vi "get remaining time budget.vi"(8 "error in":errorcluster, 10 "dt":u32=1, 11 "timing source in":refnum<class "scan engine timing source.lvclass">) -> (0 "error out":errorcluster, 2 "budget (ns)":u64, 3 "timing source out":refnum<class "scan engine timing source.lvclass">)   [LabVIEW 2013, in "scan engine timing source.lvclass"]
uses:
  scan engine timing source.lvclass
  scan engine timing source.lvclass/scan engine timing source.ctl
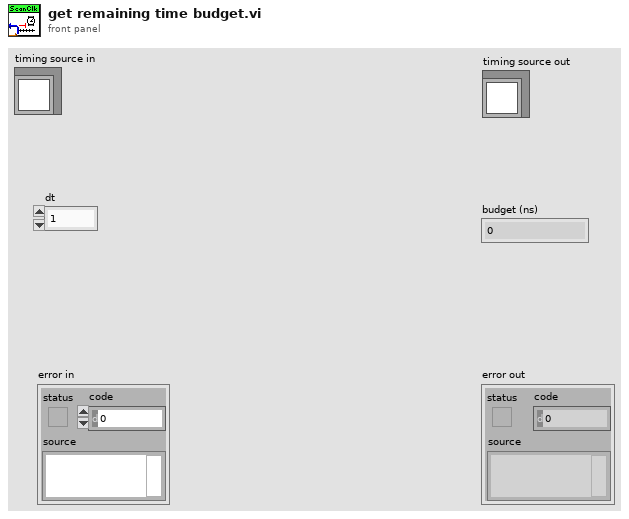
[diagram p1: front panel]
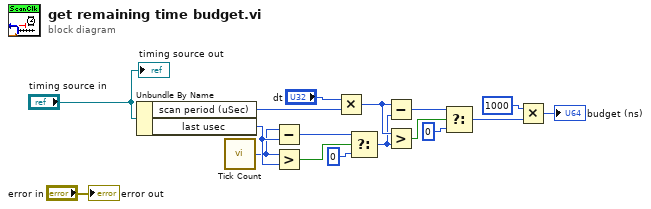
[diagram p0: block diagram]
diagram:
  n1 = Unbundle By Name("timing source in") -> ("scan period (uSec)"=w16:u32, "last usec"=w9:u32)
  n2 = call "Tick Count"() -> ("Tick Count(uSec)"=w8:u32)
  n3 = Subtract(x=w8, y=w9) -> (x-y=w11:u32)
  n4 = Greater?(x=w8, y=w9) -> (0:w12:bool)
  n5 = Multiply(x="dt", y=w16) -> (x*y=w4:u32)
  n6 = Select(t=w11, s=w12, f=u32 0) -> (s? t:f=w3:u32)
  n7 = Subtract(x=w4, y=w3) -> (x-y=w6:u32)
  n8 = Greater?(x=w4, y=w3) -> (0:w5:bool)
  n9 = Select(t=w6, s=w5, f=u32 0) -> (s? t:f=w2:u32)
  n10 = Multiply(x=u64 1000, y=w2) -> (x*y=→"budget (ns)":u64)
  "error out" <- "error in"
  "timing source out" <- "timing source in"
